vi "Get Tag SetRequest Event.vi"(6 "Namespace":string, 8 "error in (no error)":errorcluster, 10 "Tag Name":string) -> (0 "error out":errorcluster, 2 "SetRequest":refnum<user-event>)   [LabVIEW 2018, in "Tag Engine.lvlib" / "Tag Core.lvclass"]
doc: "Lookup a CVT item's set request event.\n\nIf the tag is not found, error 5602 is returned."
uses:
  Tag Core.lvclass
  Types/SetRequest Cluster.ctl
  <vilib>/Utility/Data Type/Type Definitions/Data Type.ctl
  Tag Core.lvclass/Tag Core.ctl
  Tag/Tag.lvclass/Tag.ctl
  Get Tag LUT.vi
  <vilib>/Utility/error.llb/Error Cluster From Error Code.vi
  Tag/Tag.lvclass
  Tag Engine.lvlib
  <vilib>/Utility/Data Type/NI_Data Type.lvlib
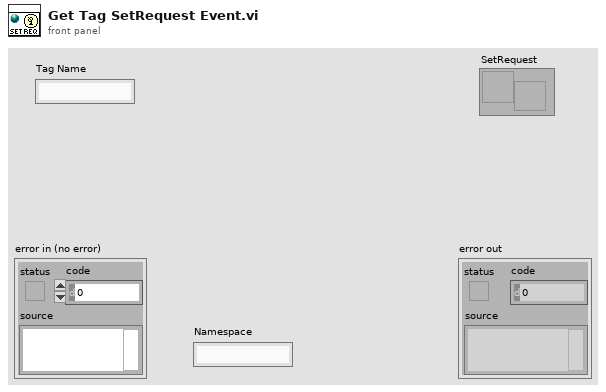
[diagram p1: front panel]
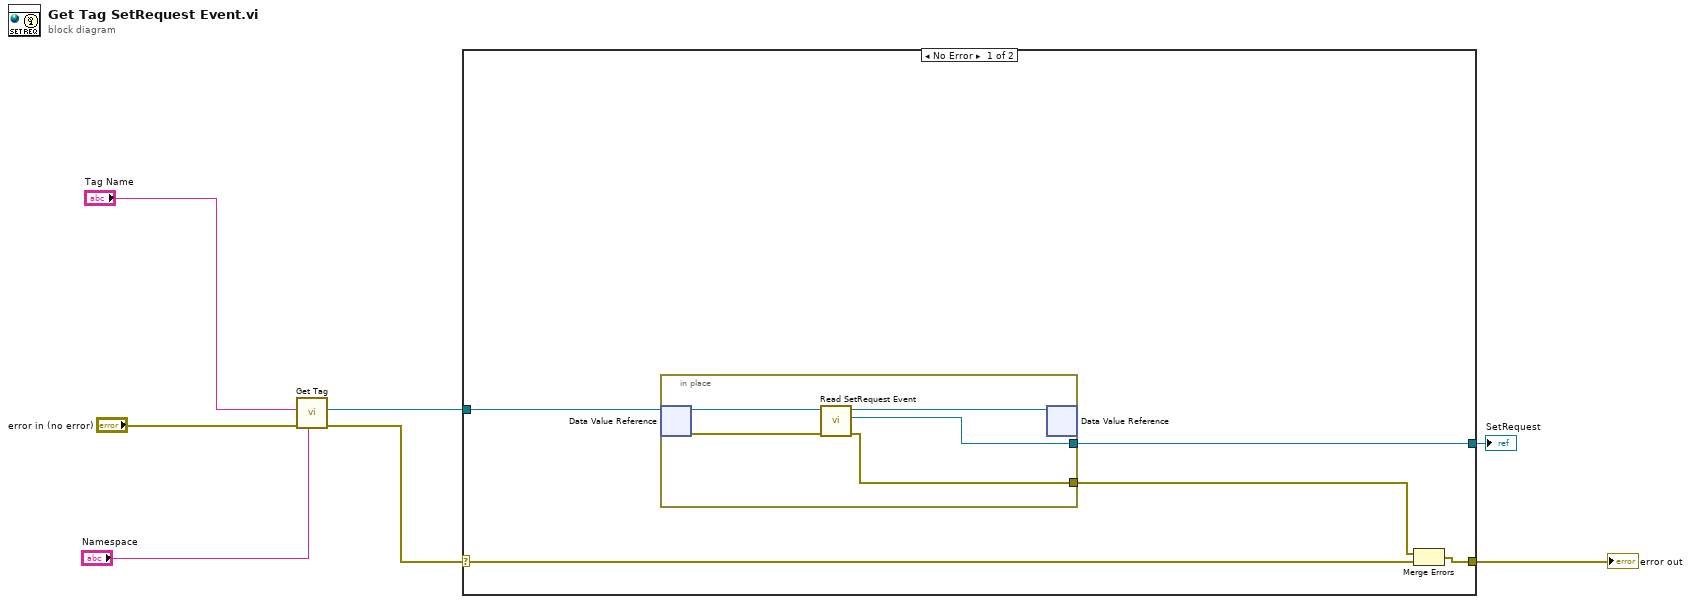
[diagram p0: block diagram]
diagram:
  n1 = call "Get Tag.vi"("Namespace"="Namespace", "error in (no error)"="error in (no error)", "Name"="Tag Name") -> ("error out"=w5:errorcluster, "Tag Ref out"=w3:refnum<data-value>)  [unwired: 6 in, 1 out]
  n2 = case shown="No Error" w5 {
    selector: w5 -> [w10 w18]
    tunnel: [w11 w18] -> w7
    tunnel: w3 -> [w12 _]
    tunnel: [w8 _] -> w2
    frame No Error {
      n3 = in-place {
        in-place-border: [w15] -> w9
        in-place-border: [w13] -> w8
        n4 = in-place-dvr #1(w12) -> (w17:refnum<class "Tag.lvclass">, w16:errorcluster)
        n5 = call "Read SetRequest Event.vi"("error in (no error)"=w16, "Tag in"=w17) -> ("error out"=w15:errorcluster, "SetRequest"=w13:refnum<user-event>, "Tag out"=w14:refnum<class "Tag.lvclass">)  [unwired: 7 in]
        n6 = in-place-dvr #1(w14) -> ()  [unwired: 2 out]
      }
      n7 = Merge Errors(w9, w10) -> (w11:errorcluster)
    }
    frame Error {
    }
  }
  "error out" <- w7
  "SetRequest" <- w2
